vi "Get Data.vi"(8 "DAQ Cluster":T1={"PSI Channel"="Dev1/ai9", "TC Channel"="Dev1/ai10", "PSI Offset"=0.555, "PSI Scale"=3000.0, "TC Offset"=1.028, "TC Scale"=144.0}, 10 "DAQ Channels In":refnum<k21>, 11 "Sim Cluster":T2) -> (2 "Temp":i32, 3 "PSI":i32)   [LabVIEW 2013]
uses:
  Controls/DAQ Cluster.ctl
  <vilib>/DAQmx/read.llb/DAQmx Read (Analog 2D DBL NChan NSamp).vi
  <vilib>/DAQmx/miscellaneous.llb/DAQmx Fill In Error Info.vi
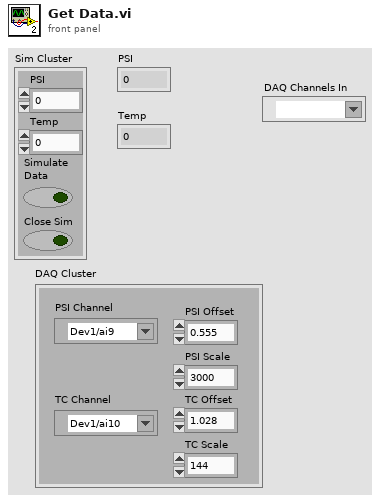
[diagram p1: front panel]
types:
  T1 = typedef "DAQ Cluster.ctl" = cluster{"PSI Channel":tag, "TC Channel":tag, "PSI Offset":dbl, "PSI Scale":dbl, "TC Offset":dbl, "TC Scale":dbl}
  T2 = cluster{"PSI":i32, "Temp":i32, "Simulate\nData":bool, "Close Sim":bool}
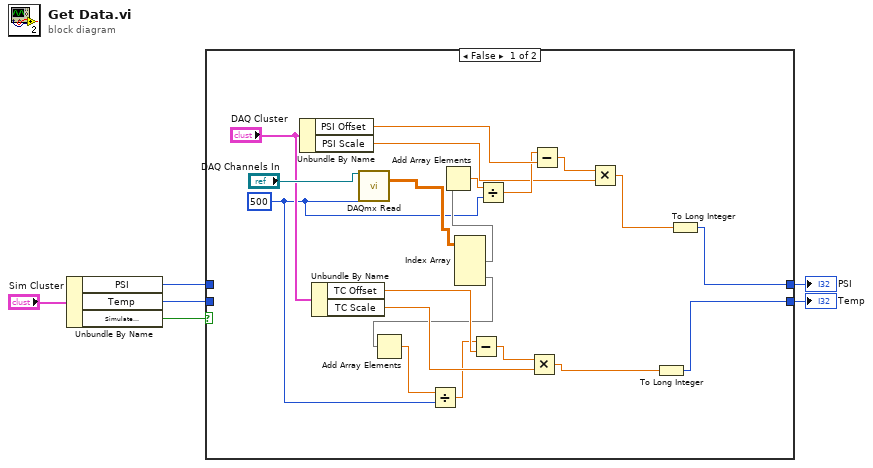
[diagram p0: block diagram]
diagram:
  n1 = Unbundle By Name("Sim Cluster") -> ("PSI"=w4:i32, "Temp"=w3:i32, "Simulate\nData"=w5:bool)
  n2 = case shown="False" w5 {
    tunnel: w4 -> [_ w28]
    tunnel: w3 -> [_ w27]
    tunnel: [w19 w28] -> w2
    tunnel: [w13 w27] -> w1
    frame False {
      w8 = 500 ("number of samples per channel")
      n3 = Unbundle By Name("DAQ Cluster") -> ("PSI Offset"=w24:dbl, "PSI Scale"=w21:dbl)
      n4 = Unbundle By Name("DAQ Cluster") -> ("TC Offset"=w16:dbl, "TC Scale"=w15:dbl)
      n5 = call-poly <vilib>:"DAQmx Read.vi"("task/channels in"="DAQ Channels In", "number of samples per channel"=w8) -> ("data"=w12:dbl[][])  [unwired: 11 in, 2 out]
      n6 = Index Array(array=w12) -> (element #1=w11:dbl[], element #2=w10:dbl[])  [unwired: 4 in]
      n7 = Add Array Elements(numeric array=w10) -> (sum=w9:dbl)
      n8 = Divide(x=w9, y=w8) -> (x/y=w7:dbl)
      n9 = Add Array Elements(numeric array=w11) -> (sum=w25:dbl)
      n10 = Subtract(x=w7, y=w16) -> (x-y=w17:dbl)
      n11 = Divide(x=w25, y=w8) -> (x/y=w23:dbl)
      n12 = Multiply(x=w17, y=w15) -> (x*y=w14:dbl)
      n13 = Subtract(x=w23, y=w24) -> (x-y=w22:dbl)
      n14 = Multiply(x=w22, y=w21) -> (x*y=w20:dbl)
      n15 = To Long Integer(number=w14) -> (32bit integer=w13:i32)
      n16 = To Long Integer(number=w20) -> (32bit integer=w19:i32)
    }
    frame True {
    }
  }
  "Temp" <- w1
  "PSI" <- w2
